vi "get-bscale.vi"() -> (0 "error out":errorcluster, 2 "bscale":dbl format="%#_9g")   [LabVIEW 2014]
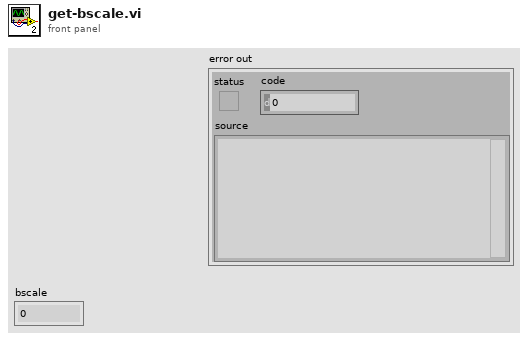
[diagram p1: front panel]
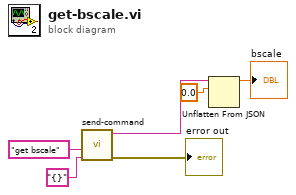
[diagram p0: block diagram]
diagram:
  n1 = call "send-command.vi"("parameters"="{}", "command"="get bscale") -> ("error out"=→"error out":errorcluster, "output"=w3:string)  [unwired: 8 in]
  n2 = Unflatten From JSON(JSON string=w3, type and defaults=0.0) -> (value=→"bscale":dbl)  [unwired: 5 in, 1 out]
